vi "setWriteFile.vi"(3 "display write dialog?":bool, 4 "append to file?":bool, 5 "file path":path) -> (0 "error out":errorcluster, 1 "Status":string="File not appended", 2 "File Refnum":refnum<file>)   [LabVIEW 2013]
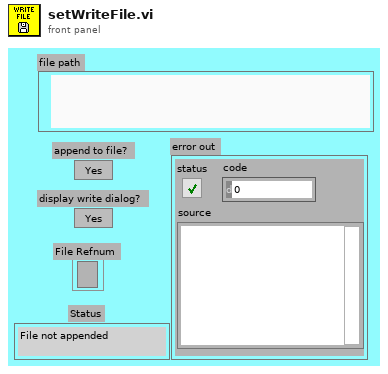
[diagram p1: front panel]
types:
  T1 = enum16{"deny read/write", "deny write-only", "deny none"}
  T2 = enum16{"open", "replace", "create", "open or create", "replace or create", "replace or create with confirmation"}
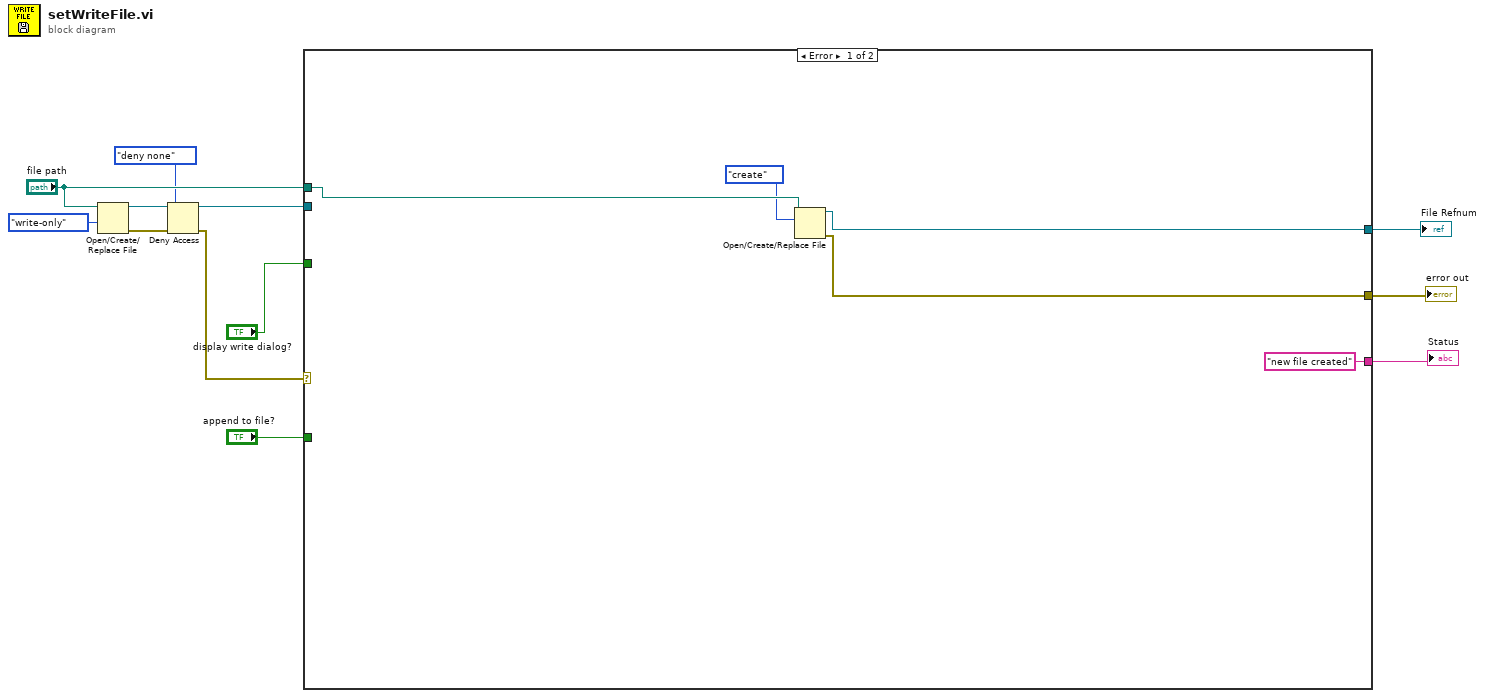
[diagram p0: block diagram]
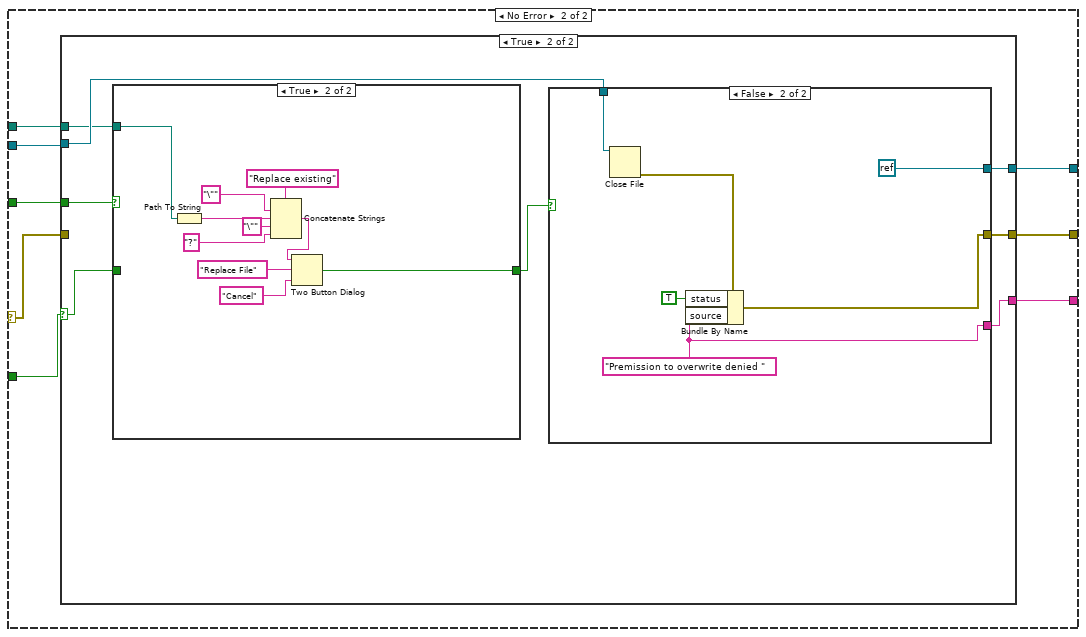
[diagram p2: hidden frame]
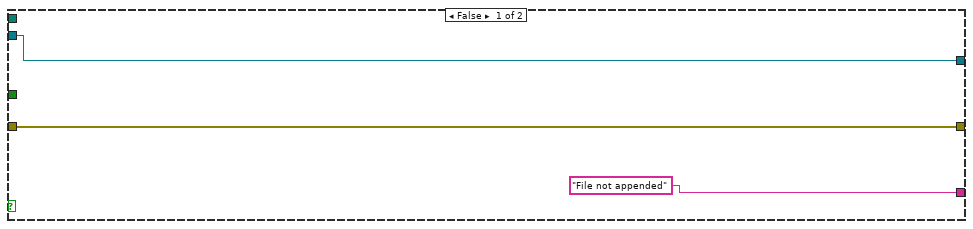
[diagram p3: hidden frame]
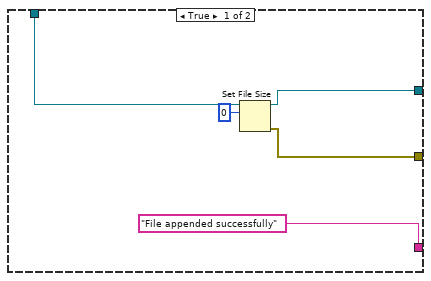
[diagram p4: hidden frame]
diagram:
  n1 = Open/Create/Replace File(file path (use dialog)="file path", access (0:read/write)=enum16{"read/write", "read-only", "write-only"}."write-only") -> (refnum out=w11:refnum<file>, error out=w4:errorcluster)  [unwired: 4 in, 1 out]
  n2 = Deny Access(4:w4, 6:T1."deny none" ("deny mode (0:deny read/write)"), 7:w11) -> (0:w2:errorcluster, 3:w3:refnum<file>)
  n3 = case shown="Error" w2 {
    selector: w2 -> [_ w19]
    tunnel: w3 -> [_ w25]
    tunnel: "file path" -> [w17 w24]
    tunnel: [w15 w23] -> w9
    tunnel: [w14 w22] -> w8
    tunnel: "append to file?" -> [_ w21]
    tunnel: "display write dialog?" -> [_ w20]
    tunnel: ["new file created" ("source") w18] -> w1
    frame Error {
      n4 = Open/Create/Replace File(file path (use dialog)=w17, operation (0:open)=T2."create") -> (refnum out=w15:refnum<file>, error out=w14:errorcluster)  [unwired: 4 in, 1 out]
    }
    frame No Error {
      n5 = case shown="True" w21 {
        selector: w21 -> [_ w30]
        tunnel: w25 -> [w28 w36]
        tunnel: w24 -> [_ w35]
        tunnel: [w28 w33] -> w23
        tunnel: [w27 w32] -> w22
        tunnel: w20 -> [_ w31]
        tunnel: w19 -> [w27 _]
        tunnel: ["File not appended" w29] -> w18
        frame False {
        }
        frame True {
          n6 = case shown="True" w31 {
            tunnel: w35 -> [_ w56]
            tunnel: [w48 w51] -> w34
            tunnel: w30 -> [w48 _]
            frame False {
            }
            frame True {
              n7 = Path To String(path=w56) -> (string=w55:string)
              n8 = Concatenate Strings("Replace existing" ("string"), "\"" ("string"), w55, "\"" ("string"), "?" ("string")) -> (w52:string)
              n9 = Two Button Dialog(message=w52, 1:"Cancel" ("T button name (\"OK\")"), 2:"Replace File" ("F button name (\"Cancel\")")) -> (T button?=w51:bool)
            }
          }
          n10 = case shown="False" w34 {
            tunnel: w36 -> [w41 w47]
            tunnel: [w39 refnum<k0> refnum] -> w33
            tunnel: [w38 w43] -> w32
            tunnel: ["File appended successfully" w42] -> w29
            frame True {
              n11 = Set File Size(6:i64 0 ("size (in bytes)"), 7:w41) -> (0:w38:errorcluster, 3:w39:refnum<file>)  [unwired: 1 in]
            }
            frame False {
              w42 = "Premission to overwrite denied " ("source")
              n12 = Close File(refnum=w47) -> (error out=w45:errorcluster)  [unwired: 1 in, 1 out]
              n13 = Bundle By Name(cluster=w45, "status"=TRUE, "source"=w42) -> (w43:errorcluster)
            }
          }
        }
      }
    }
  }
  "File Refnum" <- w9
  "error out" <- w8
  "Status" <- w1
